vi "Label Warnings List.vi"(2 "Warnings List in":string, 3 "Section":string) -> (0 "Warnings List out":string)   [LabVIEW 2013]
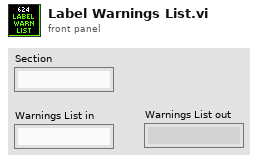
[diagram p1: front panel]
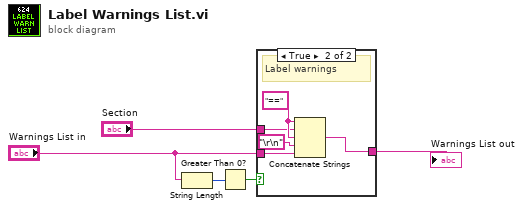
[diagram p0: block diagram]
diagram:
  n1 = String Length(string="Warnings List in") -> (length=w1:i32)
  n2 = Greater Than 0?(x=w1) -> (x > 0?=w2:bool)
  n3 = case shown="True" w2 {
    tunnel: "Warnings List in" -> [w6 w11]
    tunnel: [w6 w10] -> w4
    tunnel: "Section" -> [_ w7]
    frame False {
    }
    frame True {
      w8 = "==" ("string")
      # "Label warnings"
      n4 = Concatenate Strings(w8, w7, w8, "\r\n", w11) -> (w10:string)
    }
  }
  "Warnings List out" <- w4
